vi "Bubble Sort.vi"(8 "Sorting":T1, 11 "list in in":T2[](array[typedef]) {"Creation Date" format="%<%x>T"; "Last Updated" format="%<%x>T"}) -> (3 "list out":T2[](array[typedef]) {"Creation Date" format="%<%x>T"; "Last Updated" format="%<%x>T"})   [LabVIEW 2018]
uses:
  Type Defs/SR Cluster.ctl
  Type Defs/SR Status.ctl
  Type Defs/Sorting Methods.ctl
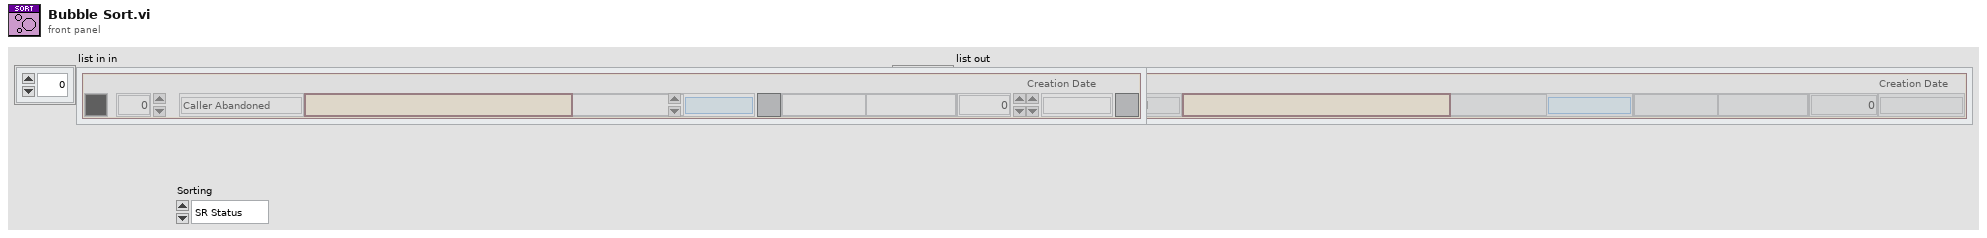
[diagram p1: front panel]
types:
  T1 = typedef "Sorting Methods.ctl" = enum16{"SR Status", "Most Recent", "SR Type", "SR Number"}
  T2 = typedef "SR Cluster.ctl" = cluster{"Color":u32, "SR Number":i32, "SR Status":T3, "Name":string, "Summary":string, "Last Updated":timestamp, "SR Type":string, "Service Level":string, "Days Open":dbl, "Creation Date":timestamp}
  T3 = typedef "SR Status.ctl" = enum16{"Caller Abandoned", "Created in Error", "Expired", "Forum Resolved AE", "Forum Resolved Customer", "IN WORK", "IN WORK Collab with AES", "IN WORK Collab with PSE", "IN WORK Collab with SE", "IN WORK Customer Added Note", "IN WORK Escalation", "IN WORK Wait on Customer", "Open", "Potentially Resolved", "Presumed Resolved", "RMA Approved for Return", "Resolved", "Passed Off"}
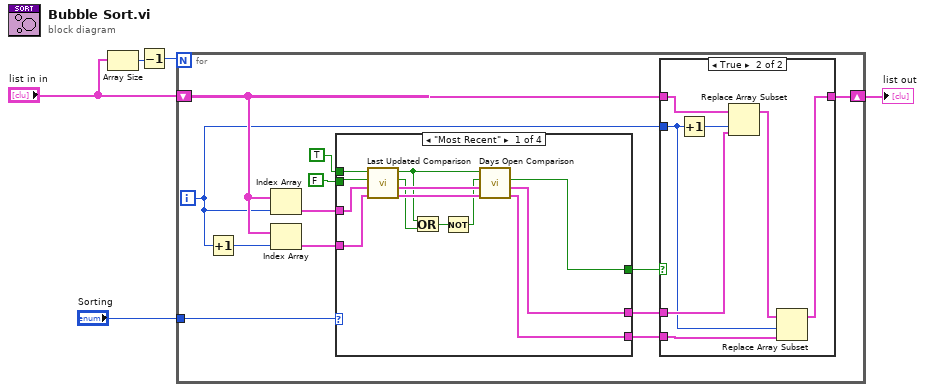
[diagram p0: block diagram]
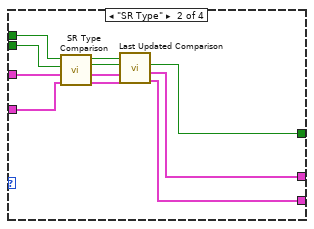
[diagram p2: hidden frame]
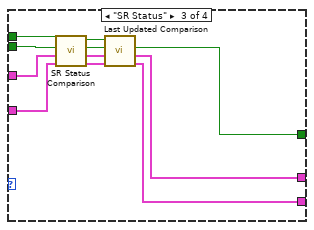
[diagram p3: hidden frame]
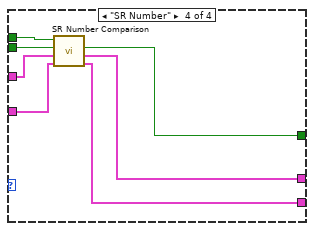
[diagram p4: hidden frame]
diagram:
  n1 = Array Size(array="list in in") -> (size(s)=w3:i32)
  n2 = Decrement(x=w3) -> (x-1=w2:i32)
  n3 = for {
    N: w2 -> [_]
    shift-right: [w13] -> w5
    shift-left: "list in in" -> [w14]
    tunnel: "Sorting" -> [w6]
    i -> [w9]
    n4 = Increment(x=w9) -> (x+1=w17:i32)
    n5 = Index Array(array=w14, index=w9) -> (element=w15:T2)
    n6 = Index Array(array=w14, index=w17) -> (element=w16:T2)
    n7 = case shown="\"Most Recent\"" w6 {
      tunnel: w16 -> [w27 w38 w49 w56]
      tunnel: w15 -> [w28 w39 w50 w57]
      tunnel: [w23 w31 w43 w54] -> w12
      tunnel: [w22 w32 w44 w53] -> w11
      tunnel: [w24 w33 w42 w55] -> w10
      tunnel: TRUE ("equal? in") -> [w30 w41 w51 w59]
      tunnel: FALSE ("flip? in") -> [w29 w40 w52 w58]
      frame "Most Recent" {
        n8 = call "Last Updated Comparison.vi"("SR Cluster 2 in"=w27, "SR Cluster 1 in"=w28, "flip? in"=w29, "equal? in"=w30) -> ("SR Cluster 2 out"=w25:T2, "SR Cluster 1 out"=w26:T2, "flip? out"=w18:bool, "equal? out"=w19:bool)  [unwired: 4 in]
        n9 = Or(x=w19, y=w18) -> (x .or. y?=w21:bool)
        n10 = Not(x=w21) -> (.not. x?=w20:bool)
        n11 = call "Days Open Comparison.vi"("SR Cluster 2 in"=w25, "SR Cluster 1 in"=w26, "flip? in"=w20, "equal? in"=w19) -> ("SR Cluster 2 out"=w22:T2, "SR Cluster 1 out"=w23:T2, "flip? out"=w24:bool)  [unwired: 4 in, 1 out]
      }
      frame "SR Type" {
        n12 = call "SR Type Comparison.vi"("SR Cluster 2 in"=w38, "SR Cluster 1 in"=w39, "flip? in"=w40, "equal? in"=w41) -> ("SR Cluster 2 out"=w37:T2, "SR Cluster 1 out"=w36:T2, "flip? out"=w35:bool, "equal? out"=w34:bool)  [unwired: 4 in]
        n13 = call "Last Updated Comparison.vi"("SR Cluster 2 in"=w37, "SR Cluster 1 in"=w36, "flip? in"=w35, "equal? in"=w34) -> ("SR Cluster 2 out"=w32:T2, "SR Cluster 1 out"=w31:T2, "flip? out"=w33:bool)  [unwired: 4 in, 1 out]
      }
      frame "SR Status" {
        n14 = call "SR Status Comparison.vi"("SR Cluster 2 in"=w49, "SR Cluster 1 in"=w50, "flip? in"=w52, "equal? in"=w51) -> ("SR Cluster 2 out"=w45:T2, "SR Cluster 1 out"=w46:T2, "flip? out"=w47:bool, "equal? out"=w48:bool)  [unwired: 4 in]
        n15 = call "Last Updated Comparison.vi"("SR Cluster 2 in"=w45, "SR Cluster 1 in"=w46, "flip? in"=w47, "equal? in"=w48) -> ("SR Cluster 2 out"=w44:T2, "SR Cluster 1 out"=w43:T2, "flip? out"=w42:bool)  [unwired: 4 in, 1 out]
      }
      frame "SR Number" {
        n16 = call "SR Number Comparison.vi"("SR Cluster 2 in"=w56, "SR Cluster 1 in"=w57, "flip? in"=w58, "equal? in"=w59) -> ("SR Cluster 2 out"=w53:T2, "SR Cluster 1 out"=w54:T2, "flip? out"=w55:bool)  [unwired: 4 in, 1 out]
      }
    }
    n17 = case shown="True" w10 {
      tunnel: w14 -> [w60 w66]
      tunnel: [w60 w61] -> w13
      tunnel: w12 -> [_ w63]
      tunnel: w11 -> [_ w65]
      tunnel: w9 -> [_ w62]
      frame False {
      }
      frame True {
        n18 = Increment(x=w62) -> (x+1=w67:i32)
        n19 = Replace Array Subset(array=w66, new element=w63, index=w67) -> (w64:T2[])
        n20 = Replace Array Subset(array=w64, new element=w65, index=w62) -> (w61:T2[])
      }
    }
  }
  "list out" <- w5
